vi "CODMn日志存储 (子VI).vi"(6 "table输入":string, 9 "参数":string, 10 "日志信息":string, 11 "database":string) -> ()   [LabVIEW 2016, in "斯坦道CODMn.lvlib"]
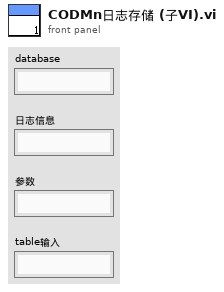
[diagram p1: front panel]
types:
  T1 = cluster{"时间标识":timestamp, "参数":string, "日志信息":string, "流程参数":string}
  T2 = cluster{"时间标识":timestamp, "设备":string, "日志信息":string, "流程参数":string}
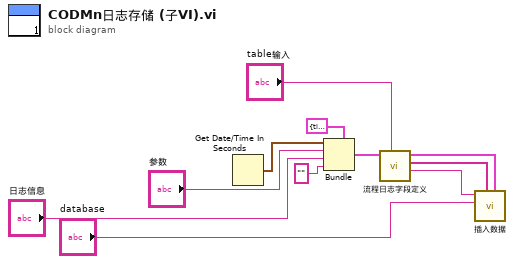
[diagram p0: block diagram]
diagram:
  n1 = Get Date/Time In Seconds() -> (seconds since 1Jan1904=w6:timestamp)
  n2 = Bundle(cluster=T1 {"时间标识"=timestamp(0 s since 1904-01-01), "参数"="", "日志信息"="", "流程参数"=""} ("data in"), "时间标识"=w6, "参数"="参数", "日志信息"="日志信息", "流程参数"="" ("table输入")) -> (w8:T1)
  n3 = call "流程日志字段定义.vi"("table输入"="table输入", "data in"=w8) -> ("table输出"=w3:string, "columns"=w2:string[], "data out"=w1:T2)  [unwired: 7 in]
  n4 = call "插入数据.vi"("data"=w1, "columns"=w2, "database"="database", "table"=w3) -> ()  [unwired: 7 in, 1 out]
